vi "gage_pressure.vi"(1 "Atmospheric Pressure [Pa]":dbl, 2 "Abs. Pressure\nVoltage [V]":dbl) -> (0 "Absolute Pressure [Pa]":dbl)   [LabVIEW 2015]
uses:
  <vilib>/express/express arith-compare/Formula/XNode/ExpressFormulaBlockNode.xnode
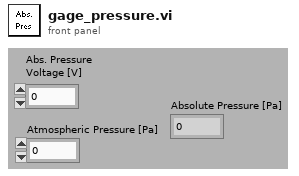
[diagram p1: front panel]
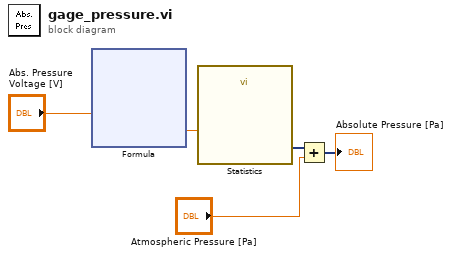
[diagram p0: block diagram]
diagram:
  n1 = xnode "Formula"("V"="Abs. Pressure\nVoltage [V]") -> ("Result"=w5:dbl)  [unwired: 1 in, 1 out]
  n2 = call "Statistics"("Signals"=w5) -> ("Arithmetic Mean"=w2:dynamicdata)  [unwired: 25 in, 1 out]
  n3 = Add(x=w2, y="Atmospheric Pressure [Pa]") -> (x+y=→"Absolute Pressure [Pa]":dynamicdata)
